vi "EncoderRead.vi"(0 "Read Encoder\n= TRUE":bool, 1 "Reset X":bool, 2 "Reset Y":bool, 3 "handle":i32, 4 "Reset  Both":bool) -> (5 "X-Encoder (mm)":dbl format="%.3f", 6 "Y-Encoder (mm)":dbl format="%.3f", 7 "X Reverse Limit":bool, 8 "X Forward Limit":bool, 9 "Y Reverse Limit":bool, 10 "Y Forward Limit":bool)   [LabVIEW 2011]
uses:
  MCL libraries/MicroDrive.dll
panel:
  out "y cur rem":i32
  out "x cur rem":i32
  out "y tot rem":i32
  out "x tot rem":i32
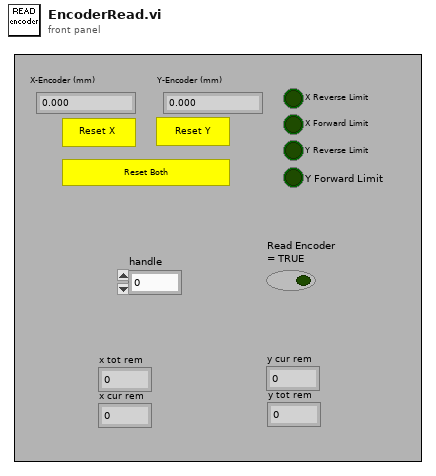
[diagram p1: front panel]
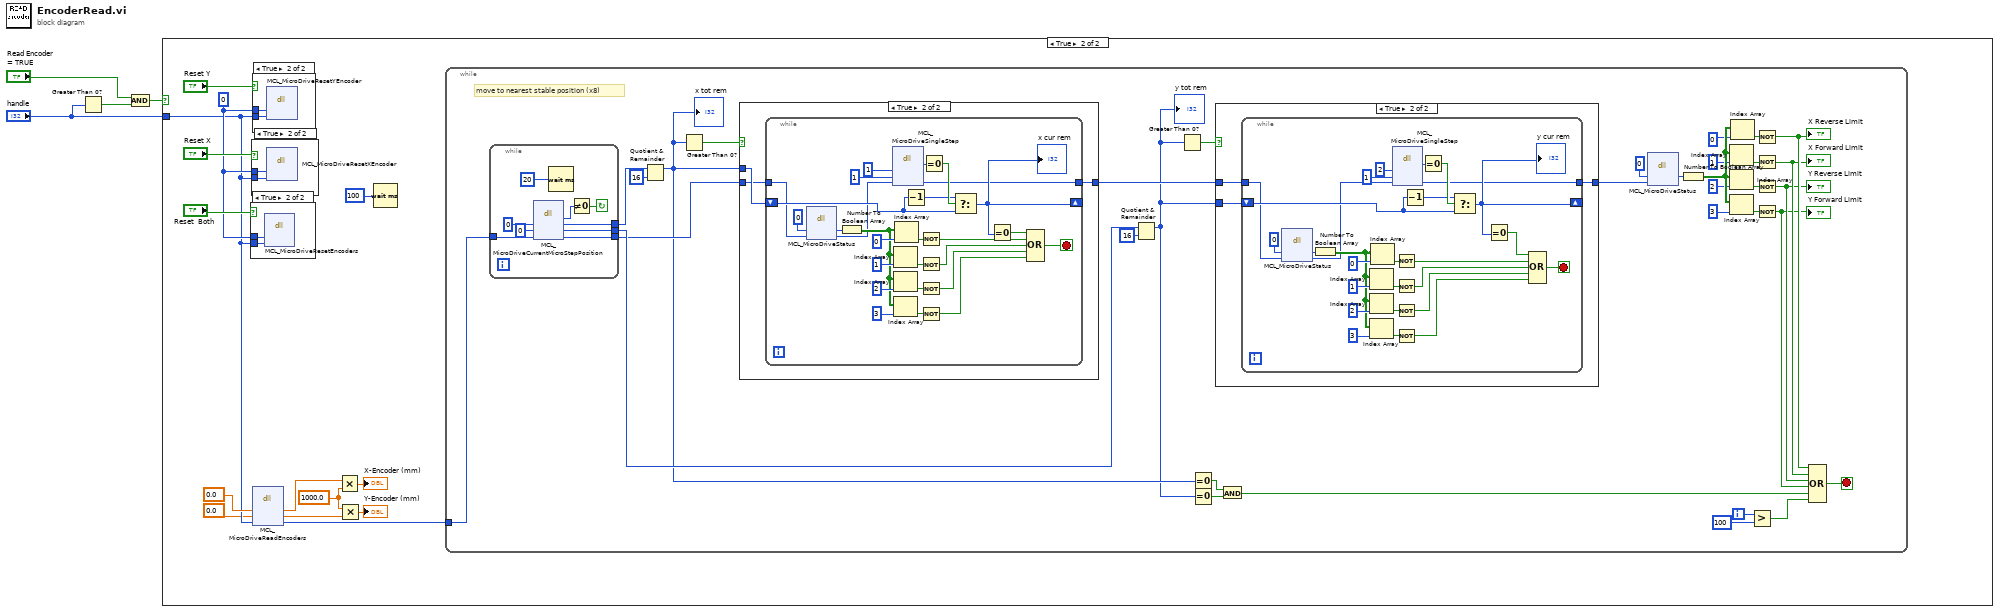
[diagram p0: block diagram]
diagram:
  n1 = Greater Than 0?(x="handle") -> (x > 0?=w1:bool)
  n2 = And(x="Read Encoder\n= TRUE", y=w1) -> (x .and. y?=w3:bool)
  n3 = case shown="True" w3 {
    tunnel: "handle" -> [_ w7]
    frame False {
    }
    frame True {
      w13 = 1000.0
      w14 = 0
      n4 = case shown="True" "Reset  Both" {
        tunnel: w14 -> [_ w127]
        tunnel: w7 -> [_ w126]
        frame False {
        }
        frame True {
          n5 = dll-call lib="F:/Vlad/Labview code/PZM_photogate/MCL libraries/MicroDrive.dll" fn="MCL_MicroDriveResetEncoders"("status"=w127, "handle"=w126) -> ()  [unwired: 4 in, 4 out]
        }
      }
      n6 = case shown="True" "Reset X" {
        tunnel: w14 -> [_ w129]
        tunnel: w7 -> [_ w128]
        frame False {
        }
        frame True {
          n7 = dll-call lib="F:/Vlad/Labview code/PZM_photogate/MCL libraries/MicroDrive.dll" fn="MCL_MicroDriveResetXEncoder"("status"=w129, "handle"=w128) -> ()  [unwired: 4 in, 4 out]
        }
      }
      n8 = case shown="True" "Reset Y" {
        tunnel: w14 -> [_ w125]
        tunnel: w7 -> [_ w124]
        frame False {
        }
        frame True {
          n9 = dll-call lib="F:/Vlad/Labview code/PZM_photogate/MCL libraries/MicroDrive.dll" fn="MCL_MicroDriveResetYEncoder"("status"=w125, "handle"=w124) -> ()  [unwired: 4 in, 4 out]
        }
      }
      n10 = dll-call lib="F:/Vlad/Labview code/PZM_photogate/MCL libraries/MicroDrive.dll" fn="MCL_MicroDriveReadEncoders"("xenc"=0.0, "yenc"=0.0, "handle"=w7) -> ("xenc"=w12:dbl, "yenc"=w11:dbl, "handle"=w5:i32)  [unwired: 3 in, 3 out]
      n11 = Multiply(x=w12, y=w13) -> (x*y=→"X-Encoder (mm)":dbl)
      n12 = Multiply(x=w13, y=w11) -> (x*y=→"Y-Encoder (mm)":dbl)
      n13 = Wait (ms)(milliseconds to wait=100) -> ()  [unwired: 1 out]
      n14 = while {
        tunnel: w5 -> [w52]
        i -> [w21]
        stop <- w22 stop-if-true
        # "move to nearest stable position (x8)"
        n15 = while {
          tunnel: w52 -> [w61]
          tunnel: [w58] -> w51
          tunnel: [w57] -> w45
          tunnel: [w56] -> w44
          stop <- w55 continue-if-true
          n16 = dll-call lib="F:/Vlad/Labview code/PZM_photogate/MCL libraries/MicroDrive.dll" fn="MCL_MicroDriveCurrentMicroStepPosition"("microStepsX"=0, "microStepsY"=0, "handle"=w61) -> ("MCL_SUCCESS"=w54:i32, "microStepsX"=w58:i32, "microStepsY"=w57:i32, "handle"=w56:i32)  [unwired: 3 in, 2 out]
          n17 = Wait (ms)(milliseconds to wait=20) -> ()  [unwired: 1 out]
          n18 = Not Equal To 0?(x=w54) -> (x != 0?=w55:bool)
        }
        n19 = Quotient & Remainder(x=w51, y=16) -> (x-y*floor(x/y)=w41:i32)  [unwired: 1 out]
        "x tot rem" <- w41
        n20 = Greater Than 0?(x=w41) -> (x > 0?=w48:bool)
        n21 = case shown="True" w48 {
          tunnel: w41 -> [_ w96]
          tunnel: w44 -> [w93 w95]
          tunnel: [w93 w94] -> w46
          frame False {
          }
          frame True {
            n22 = while {
              tunnel: w95 -> [w98]
              shift-right: [w116] -> _
              shift-left: w96 -> [w119]
              tunnel: [w115] -> w94
              stop <- w103 stop-if-true
              n23 = dll-call lib="F:/Vlad/Labview code/PZM_photogate/MCL libraries/MicroDrive.dll" fn="MCL_MicroDriveStatus"("status"=0, "handle"=w98) -> ("status"=w105:u8, "handle"=w97:i32)  [unwired: 3 in, 3 out]
              n24 = Number To Boolean Array(number=w105) -> (Boolean array=w106:bool[])
              n25 = dll-call lib="F:/Vlad/Labview code/PZM_photogate/MCL libraries/MicroDrive.dll" fn="MCL_MicroDriveSingleStep"("axis"=u32 1, "direction"=1, "handle"=w97) -> ("MCL_SUCCESS"=w121:i32, "handle"=w115:i32)  [unwired: 5 in, 2 out]
              n26 = Index Array(array=w106, index=1) -> (element=w113:bool)
              n27 = Index Array(array=w106, index=2) -> (element=w112:bool)
              n28 = Index Array(array=w106, index=3) -> (element=w111:bool)
              n29 = Index Array(array=w106, index=0) -> (element=w114:bool)
              n30 = Decrement(x=w119) -> (x-1=w118:i32)
              n31 = Not(x=w114) -> (.not. x?=w102:bool)
              n32 = Not(x=w113) -> (.not. x?=w101:bool)
              n33 = Not(x=w112) -> (.not. x?=w100:bool)
              n34 = Not(x=w111) -> (.not. x?=w99:bool)
              n35 = Equal To 0?(x=w121) -> (x = 0?=w120:bool)
              n36 = Select(t=w118, s=w120, f=w119) -> (s? t:f=w116:i32)
              "x cur rem" <- w116
              n37 = Equal To 0?(x=w116) -> (x = 0?=w117:bool)
              n38 = Compound Arithmetic op=OR(w117, w102, w101, w100, w99) -> (w103:bool)
            }
          }
        }
        n39 = Quotient & Remainder(x=w45, y=16) -> (x-y*floor(x/y)=w40:i32)  [unwired: 1 out]
        "y tot rem" <- w40
        n40 = Greater Than 0?(x=w40) -> (x > 0?=w47:bool)
        n41 = Equal To 0?(x=w41) -> (x = 0?=w43:bool)
        n42 = Equal To 0?(x=w40) -> (x = 0?=w42:bool)
        n43 = case shown="True" w47 {
          tunnel: w40 -> [_ w65]
          tunnel: w46 -> [w62 w64]
          tunnel: [w62 w63] -> w28
          frame False {
          }
          frame True {
            n44 = while {
              tunnel: w64 -> [w69]
              shift-right: [w86] -> _
              shift-left: w65 -> [w88]
              tunnel: [w85] -> w63
              stop <- w66 stop-if-true
              n45 = dll-call lib="F:/Vlad/Labview code/PZM_photogate/MCL libraries/MicroDrive.dll" fn="MCL_MicroDriveStatus"("status"=0, "handle"=w69) -> ("status"=w80:u8, "handle"=w68:i32)  [unwired: 3 in, 3 out]
              n46 = Number To Boolean Array(number=w80) -> (Boolean array=w72:bool[])
              n47 = Index Array(array=w72, index=1) -> (element=w73:bool)
              n48 = Index Array(array=w72, index=2) -> (element=w74:bool)
              n49 = Index Array(array=w72, index=3) -> (element=w75:bool)
              n50 = Index Array(array=w72, index=0) -> (element=w71:bool)
              n51 = dll-call lib="F:/Vlad/Labview code/PZM_photogate/MCL libraries/MicroDrive.dll" fn="MCL_MicroDriveSingleStep"("axis"=u32 2, "direction"=1, "handle"=w68) -> ("MCL_SUCCESS"=w90:i32, "handle"=w85:i32)  [unwired: 5 in, 2 out]
              n52 = Not(x=w71) -> (.not. x?=w81:bool)
              n53 = Not(x=w73) -> (.not. x?=w82:bool)
              n54 = Not(x=w74) -> (.not. x?=w83:bool)
              n55 = Not(x=w75) -> (.not. x?=w84:bool)
              n56 = Decrement(x=w88) -> (x-1=w87:i32)
              n57 = Equal To 0?(x=w90) -> (x = 0?=w89:bool)
              n58 = Select(t=w87, s=w89, f=w88) -> (s? t:f=w86:i32)
              "y cur rem" <- w86
              n59 = Equal To 0?(x=w86) -> (x = 0?=w67:bool)
              n60 = Compound Arithmetic op=OR(w67, w81, w82, w83, w84) -> (w66:bool)
            }
          }
        }
        n61 = And(x=w43, y=w42) -> (x .and. y?=w23:bool)
        n62 = dll-call lib="F:/Vlad/Labview code/PZM_photogate/MCL libraries/MicroDrive.dll" fn="MCL_MicroDriveStatus"("status"=0, "handle"=w28) -> ("status"=w38:u8)  [unwired: 4 in, 3 out]
        n63 = Number To Boolean Array(number=w38) -> (Boolean array=w37:bool[])
        n64 = Index Array(array=w37, index=1) -> (element=w30:bool)
        n65 = Index Array(array=w37, index=2) -> (element=w31:bool)
        n66 = Index Array(array=w37, index=3) -> (element=w32:bool)
        n67 = Index Array(array=w37, index=0) -> (element=w29:bool)
        n68 = Greater?(x=w21, y=100) -> (0:w19:bool)
        n69 = Not(x=w29) -> (.not. x?=w27:bool)
        "X Reverse Limit" <- w27
        n70 = Not(x=w30) -> (.not. x?=w26:bool)
        "X Forward Limit" <- w26
        n71 = Not(x=w31) -> (.not. x?=w25:bool)
        "Y Reverse Limit" <- w25
        n72 = Not(x=w32) -> (.not. x?=w24:bool)
        "Y Forward Limit" <- w24
        n73 = Compound Arithmetic op=OR(w27, w26, w25, w24, w23, w19) -> (w22:bool)
      }
    }
  }
